vi "Add.vi"(8 "error in (no error)":errorcluster, 9 "uService":string, 10 "Guardian":string, 11 "Distr uS Map ref in":refnum<data-value>) -> (0 "error out":errorcluster, 2 "List unchanged?":bool, 3 "Distr uS Map ref out":refnum<data-value>)   [LabVIEW 2026, in "TALOS.lvlib" / "Classes.lvlib" / "Distributed uService Map.lvclass"]
uses:
  Distributed uService Map.lvclass
  Distributed uService Map.lvclass/Distributed uService Map.ctl
  Ancestor/Ancestor/Ancestor.lvclass/Ancestor.ctl
  Support VIs/Generate Error.vi
  FGV/Error Memory/Get Error Description.vi
  Support VIs/Get PC name.vi
  Ancestor/Ancestor/Read ID.vi
  Support VIs/Get Class Name.vi
  <vilib>/Utility/error.llb/Clear Errors.vi
  FGV/Error Memory/Error Memory Core.vi
  <vilib>/AdvancedString/Delimited String to 1D String Array.vi
  <vilib>/AdvancedString/Delimited String to 1D String Array (string).vi
  Support VIs/Circus Root Path.vi
  FGV/Error Memory/Error Crt Lvl checker.vi
  FGV/Error Memory/Error Memory Core.vi/40c8088d-b597-4017-91af-faa98e00292e.vi
  FGV/Error Memory/Error Memory Core.vi/d4a3ab98-063c-4e44-b43d-fbdcfe6c2be2.vi
  Support VIs/Global Memory.vi
  <vilib>/Utility/LVClass/Get LV Class Name.vi
  Support VIs/Is in Packed Library.vi
  Support VIs/TALOS Root path.vi
  Support VIs/Read CSV worksheet.vi
  Support VIs/Global Constants.vi
  <vilib>/Utility/error.llb/General Error Handler.vi
  Support VIs/Error Log.vi
  Ancestor/Ancestor/Ancestor.lvclass
  <vilib>/Comparison/Equal/Equal Functor/Equal Functor.lvclass
  TALOS.lvlib
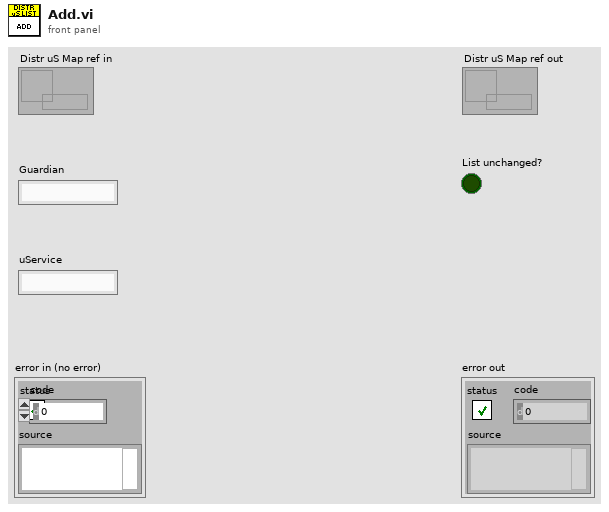
[diagram p1: front panel]
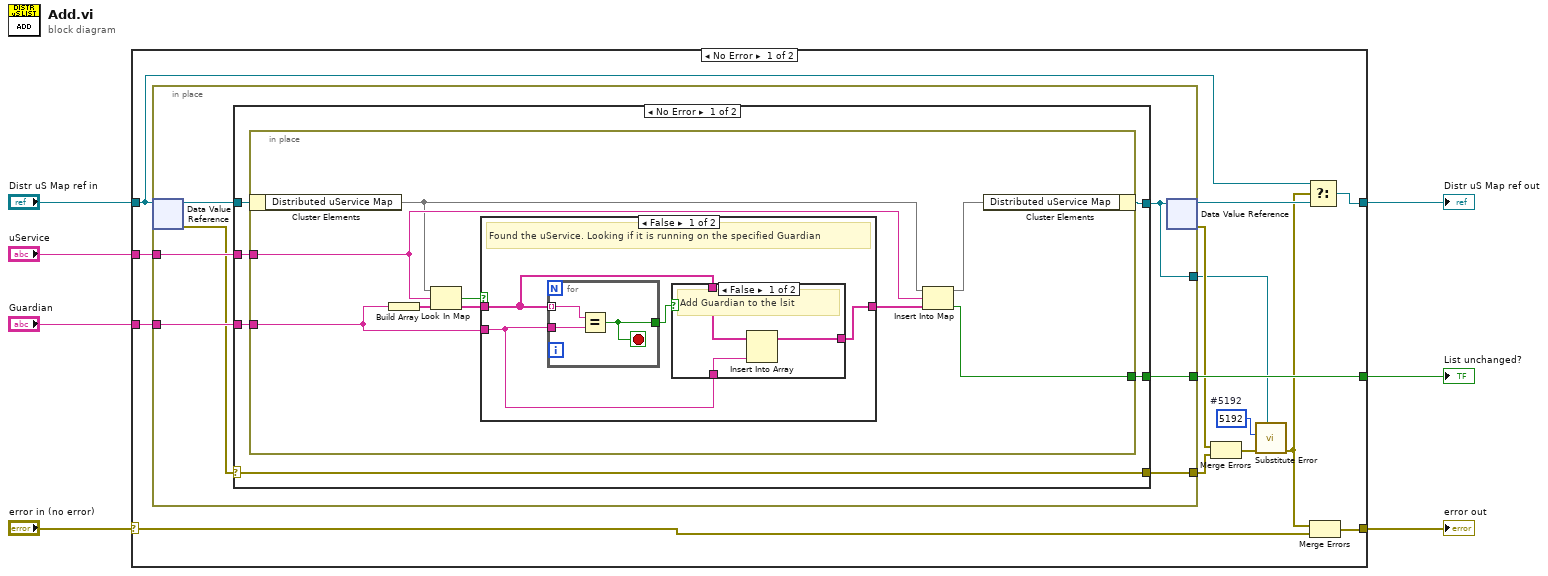
[diagram p0: block diagram]
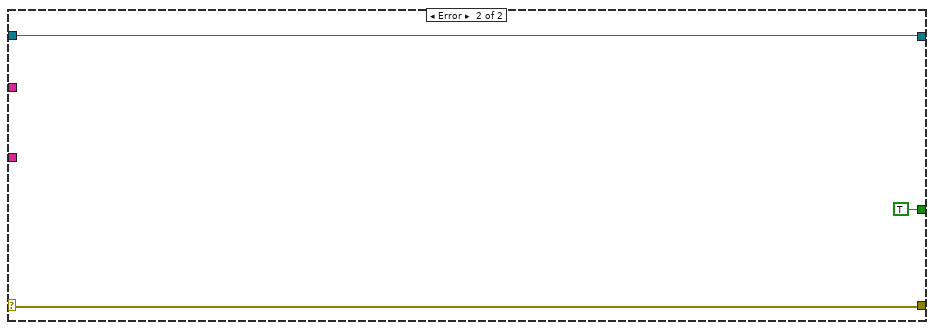
[diagram p4: hidden frame]
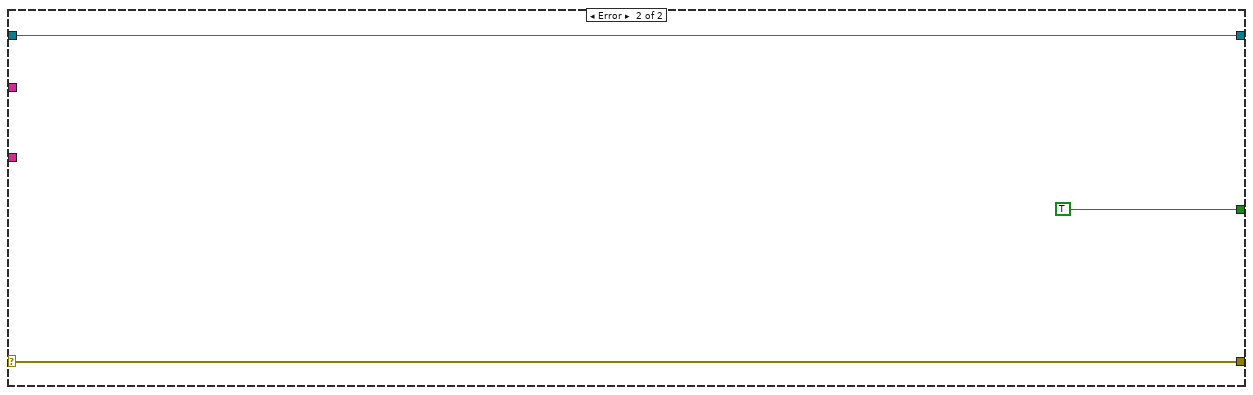
[diagram p5: hidden frame]
diagram:
  n1 = case shown="No Error" "error in (no error)" {
    selector: "error in (no error)" -> [w14 w60]
    tunnel: [w15 w60] -> w6
    tunnel: "uService" -> [w21 _]
    tunnel: "Guardian" -> [w20 _]
    tunnel: [w19 TRUE ("value unchanged?")] -> w3
    tunnel: "Distr uS Map ref in" -> [w17 w61]
    tunnel: [w16 w61] -> w1
    frame No Error {
      w11 = 5192  # #5192
      n2 = in-place {
        in-place-border: [w28] -> w13
        in-place-border: w21 -> [w27]
        in-place-border: w20 -> [w26]
        in-place-border: [w25] -> w19
        in-place-border: [w22] -> w9
        n3 = in-place-dvr #1(w17) -> (w24:refnum<class "Distributed uService Map.lvclass">, w23:errorcluster)
        n4 = case shown="No Error" w23 {
          selector: w23 -> [w34 w56]
          tunnel: [w34 w56] -> w28
          tunnel: [w30 w57] -> w22
          tunnel: w27 -> [w32 _]
          tunnel: w26 -> [w33 _]
          tunnel: [w31 TRUE ("value unchanged?")] -> w25
          tunnel: w24 -> [w29 w57]
          frame No Error {
            n5 = in-place {
              in-place-border: w33 -> [w40]
              in-place-border: w32 -> [w39]
              in-place-border: [w37] -> w31
              n6 = in-place-cluster #2(w29) -> ("Distributed uService Map"=w35:map{string, string[]})
              n7 = Build Array(w40) -> (w41:string[])
              n8 = Look In Map(map=w35, key=w39, default value=w41) -> (key not found?=w43:bool, value=w42:string[])
              n9 = case shown="False" w43 {
                tunnel: w42 -> [w44 w55]
                tunnel: [w45 w55] -> w38
                tunnel: w40 -> [w46 _]
                frame False {
                  # "Found the uService. Looking if it is running on the specified Guardian"
                  n10 = for {
                    tunnel: w44 -> [w49] mode=indexing
                    tunnel: w46 -> [w50]
                    tunnel: [w48] -> w47
                    stop <- w48 stop-if-true
                    n11 = Equal?(x=w49, y=w50) -> (x = y?=w48:bool)
                  }
                  n12 = case shown="False" w47 {
                    tunnel: w44 -> [w53 w54]
                    tunnel: [w51 w54] -> w45
                    tunnel: w46 -> [w52 _]
                    frame False {
                      # "Add Guardian to the lsit"
                      n13 = Insert Into Array(array=w53, new element=w52) -> (w51:string[])  [unwired: 1 in]
                    }
                    frame True {
                      # "The uService is running already"
                    }
                  }
                }
                frame True {
                  # "There is no other instance of the uService running"
                }
              }
              n14 = Insert Into Map(map in=w35, key=w39, value=w38) -> (map out=w36:map{string, string[]}, value unchanged?=w37:bool)  [unwired: 1 out]
              n15 = in-place-cluster #2("Distributed uService Map"=w36) -> (w30:refnum<class "Distributed uService Map.lvclass">)
            }
          }
          frame Error {
          }
        }
        n16 = in-place-dvr #1(w22) -> (w18:refnum<data-value>, w12:errorcluster)
      }
      n17 = Merge Errors(w12, w13) -> (w10:errorcluster)
      n18 = call "Substitute Error.vi"("LabVIEW Object"=w9, "error in (no error)"=w10, "Error Code"=w11) -> ("error out"=w8:errorcluster)  [unwired: 8 in]
      n19 = Select(t=w17, s=w8, f=w18) -> (s? t:f=w16:refnum<data-value>)
      n20 = Merge Errors(w8, w14) -> (w15:errorcluster)
    }
    frame Error {
    }
  }
  "error out" <- w6
  "List unchanged?" <- w3
  "Distr uS Map ref out" <- w1
